vi "SIC_Query.vi"(0 "System no.":i32=1 min=1 max=4 step=1, 2 "Analog input IDs":i32[](array[numeric]) min=1 max=10 step=1, 3 "All inputs?":bool, 5 "error in":errorcluster) -> (14 "Analog input IDs out":i32[](array[numeric]) min=1 max=10 step=1, 15 "Signal input calculation type":i32[](array[numeric]), 16 "Signal input calculation parameters":dbl[][](array[numeric]), 19 "error out":errorcluster)   [LabVIEW 2020]
doc: "Query Fast alignment Input Calculation\n\nSignal input calculation Type:\n0 = Calculation OFF\n1 = Exponential Calculation: \nCalculated Input Signal = Parameter0 + Parameter1 * Parameter2^(Parameter3*Voltage)\n2 = Polynomial Calculation:\n Calculated Input Signal = Parameter0 + Parameter1*Voltage^1 + Parameter2*Voltage^2 + Parameter3*Voltage^3 + Parameter4*Voltage^4)\n\n\nC-887, E-712: \nE-727: Only calculation type 0 supported."
uses:
  whitespace.ctl
panel:
  # "Query Fast alignment Input Calculation"
  # "Query"
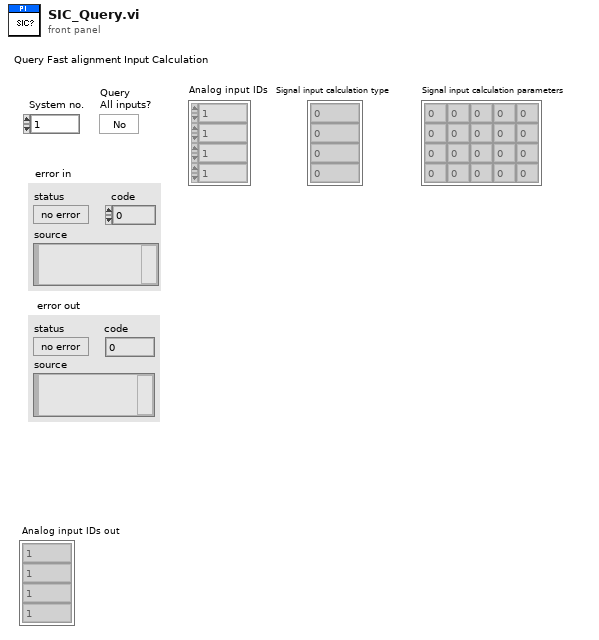
[diagram p1: front panel]
types:
  T1 = typedef "whitespace.ctl" = u16
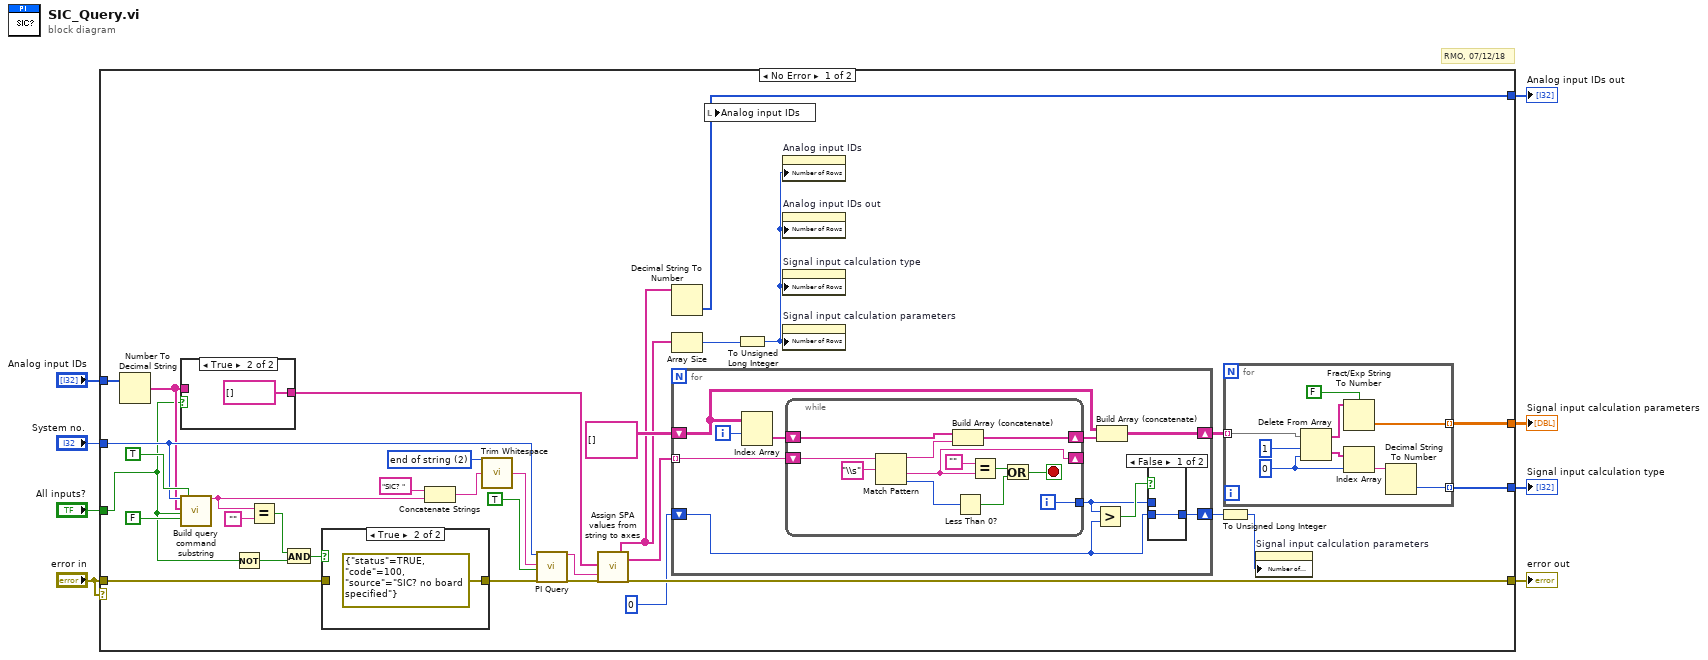
[diagram p0: block diagram]
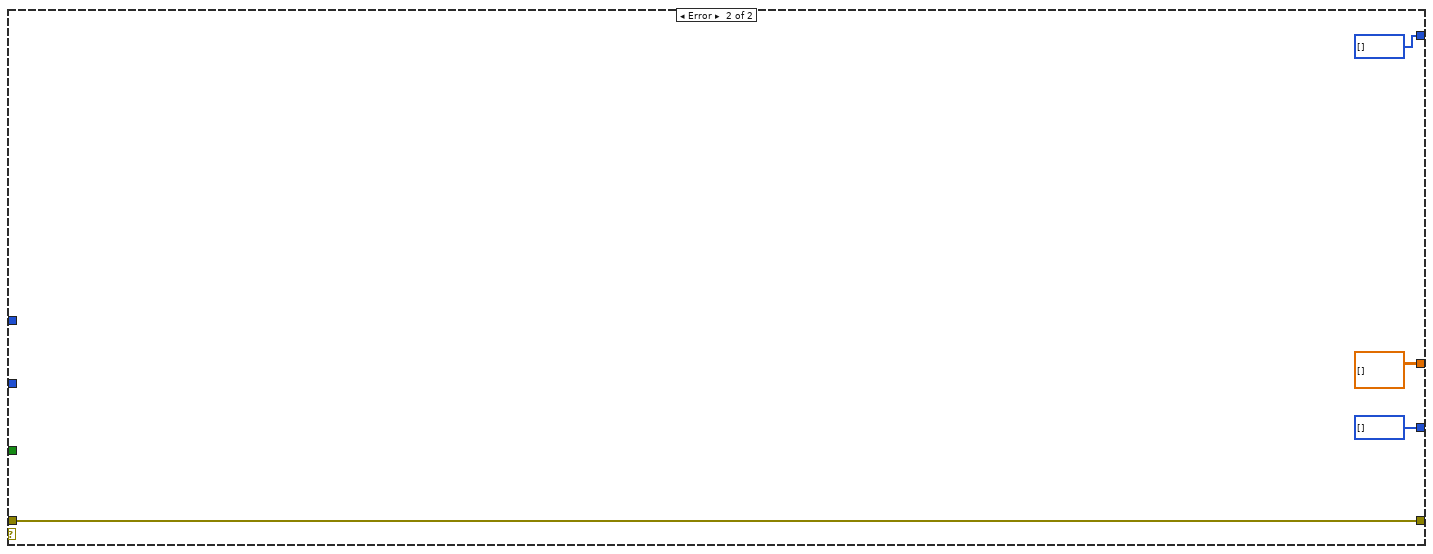
[diagram p5: hidden frame]
diagram:
  # "RMO, 07/12/18"
  n1 = case shown="No Error" "error in" {
    tunnel: "error in" -> [w33 w83]
    tunnel: "Analog input IDs" -> [w24 _]
    tunnel: [w29 w83] -> w7
    tunnel: "System no." -> [w30 _]
    tunnel: "All inputs?" -> [w19 _]
    tunnel: [w22 i32[] []] -> w4
    tunnel: [w17 dbl[][] []] -> w3
    tunnel: [w16 i32[] []] -> w2
    frame No Error {
      w11 = T1 2 items=["both", "start of string", "end of string"] ("location (both)")
      n2 = Number To Decimal String(number=w24) -> (decimal integer string=w21:string[])  [unwired: 1 out]
      n3 = case shown="True" w19 {
        tunnel: w21 -> [w52 _]
        tunnel: [w52 string[] []] -> w20
        frame False {
        }
        frame True {
        }
      }
      n4 = call "Build query command substring.vi"("System no."=w30, "Axes to query in"=w21, "Query\nAll axes?"=w19, "For all axes: use\nAxis identifier?"=FALSE ("For all axes: use\nAxis identifier?"), "With space?"=TRUE) -> ("Command substring"=w38:string)  [unwired: 1 in, 13 out]
      n5 = Not(x=w19) -> (.not. x?=w36:bool)
      n6 = Equal?(x=w38, y="" ("x")) -> (x = y?=w37:bool)
      n7 = And(x=w37, y=w36) -> (x .and. y?=w39:bool)
      n8 = case shown="True" w39 {
        tunnel: [w78 errorcluster {"status"=TRUE, "code"=100, "source"="SIC? no board specified"} ("error out")] -> w32
        tunnel: w33 -> [w78 _]
        frame False {
        }
        frame True {
        }
      }
      n9 = Concatenate Strings("SIC? ", w38) -> (w13:string)
      n10 = call "Trim Whitespace.vi"("string"=w13, "location (both)"=w11) -> ("trimmed string"=w12:string)
      n11 = call "PI Query.vi"("System no."=w30, "String to send"=w12, "Attach termination char.?"=TRUE ("Attach Linefeed?"), "error in"=w32) -> ("String read"=w9:string, "error out"=w10:errorcluster)  [unwired: 3 in, 11 out]
      n12 = call "Assign SPA values from string to axes.vi"("Queried axes"=w20, "Input string"=w9, "error in"=w10) -> ("Queried axes out"=w23:string[], "Parameter strings"=w28:string[], "error out"=w29:errorcluster)  [unwired: 4 in, 10 out]
      n13 = Decimal String To Number(string=w23) -> (number=w22:i32[])  [unwired: 3 out]
      n14 = Array Size(array=w23) -> (size(s)=w27:i32)
      n15 = for {
        tunnel: w28 -> [w63] mode=indexing
        shift-right: [w62] -> w18
        shift-left: string[][] [] -> [w60]
        shift-right: [w55] -> w25
        shift-left: 0 -> [w54]
        i -> [w59]
        n16 = Index Array(array=w60, index (row)=w59) -> (element=w58:string[])  [unwired: 1 in]
        n17 = while {
          shift-right: [w73] -> w61
          shift-left: w58 -> [w75]
          shift-right: [w71] -> _
          shift-left: w63 -> [w77]
          tunnel: [w66] -> w56
          i -> [w66]
          stop <- w68 stop-if-true
          n18 = Match Pattern(string=w77, regular expression="\\s") -> (before substring=w74:string, after substring=w71:string, offset past match=w72:i32)  [unwired: 2 out]
          n19 = Build Array (concatenate)(w75, w74) -> (w73:string[])
          n20 = Less Than 0?(x=w72) -> (x < 0?=w69:bool)
          n21 = Equal?(x="", y=w71) -> (x = y?=w67:bool)
          n22 = Or(x=w67, y=w69) -> (x .or. y?=w68:bool)
        }
        n23 = Greater?(x=w56, y=w54) -> (0:w57:bool)
        n24 = Build Array (concatenate)(w60, w61) -> (w62:string[][])
        n25 = case shown="False" w57 {
          tunnel: w56 -> [_ w65]
          tunnel: [w64 w65] -> w55
          tunnel: w54 -> [w64 _]
          frame False {
          }
          frame True {
          }
        }
      }
      n26 = local write "Analog input IDs"(w22) -> ()
      n27 = To Unsigned Long Integer(number=w27) -> (unsigned 32bit integer=w14:u32)
      n28 = property on="Analog input IDs" class="Arr (strict)"("Number of Rows"=w14) -> ()  [unwired: 2 in, 2 out]
      n29 = property on="Analog input IDs out" class="Arr (strict)"("Number of Rows"=w14) -> ()  [unwired: 2 in, 2 out]
      n30 = property on="Signal input calculation type" class="Arr (strict)"("Number of Rows"=w14) -> ()  [unwired: 2 in, 2 out]
      n31 = property on="Signal input calculation parameters" class="Arr (strict)"("Number of Rows"=w14) -> ()  [unwired: 2 in, 2 out]
      n32 = To Unsigned Long Integer(number=w25) -> (unsigned 32bit integer=w15:u32)
      n33 = for {
        tunnel: w18 -> [w51] mode=indexing
        tunnel: [w49] -> w16 mode=indexing
        tunnel: [w46] -> w17 mode=indexing
        w43 = 0
        n34 = Delete From Array(array=w51, length=1, index=w43) -> (deleted portion=w45:string[], array with subset deleted=w48:string[])
        n35 = Fract/Exp String To Number(use system decimal point (T)=FALSE, string=w48) -> (number=w46:dbl[])  [unwired: 3 out]
        n36 = Index Array(array=w45, index=w43) -> (element=w44:string)
        n37 = Decimal String To Number(string=w44) -> (number=w49:i32)  [unwired: 3 out]
      }
      n38 = property on="Signal input calculation parameters" class="Arr (strict)"("Number of Columns"=w15) -> ()  [unwired: 2 in, 2 out]
    }
    frame Error {
    }
  }
  "error out" <- w7
  "Analog input IDs out" <- w4
  "Signal input calculation parameters" <- w3
  "Signal input calculation type" <- w2
